vi "ihm_conv.vi"() -> ()   [LabVIEW 2014]
panel:
  out "out path":path
  out "nbrCmd":i32
  out "Array 2":u8[][](array[numeric]) format="%.0x"
  out "Numeric":i32
  out "length":i32
  out "reste":string
  out "parametre":string
  out "commande":string
  out "Lettre":string
  out "appended path":path
  out "text":string
  out "Array":string[](array[string])
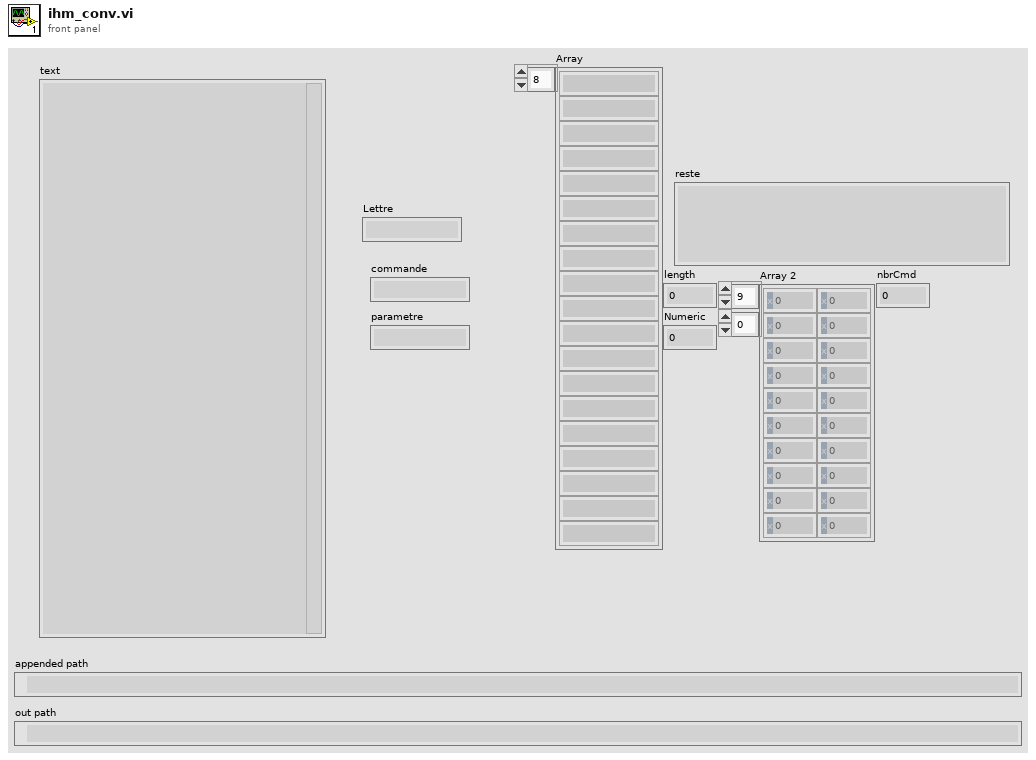
[diagram p1: front panel]
types:
  T1 = enum16{"open", "replace", "create", "open or create", "replace or create", "replace or create with confirmation"}
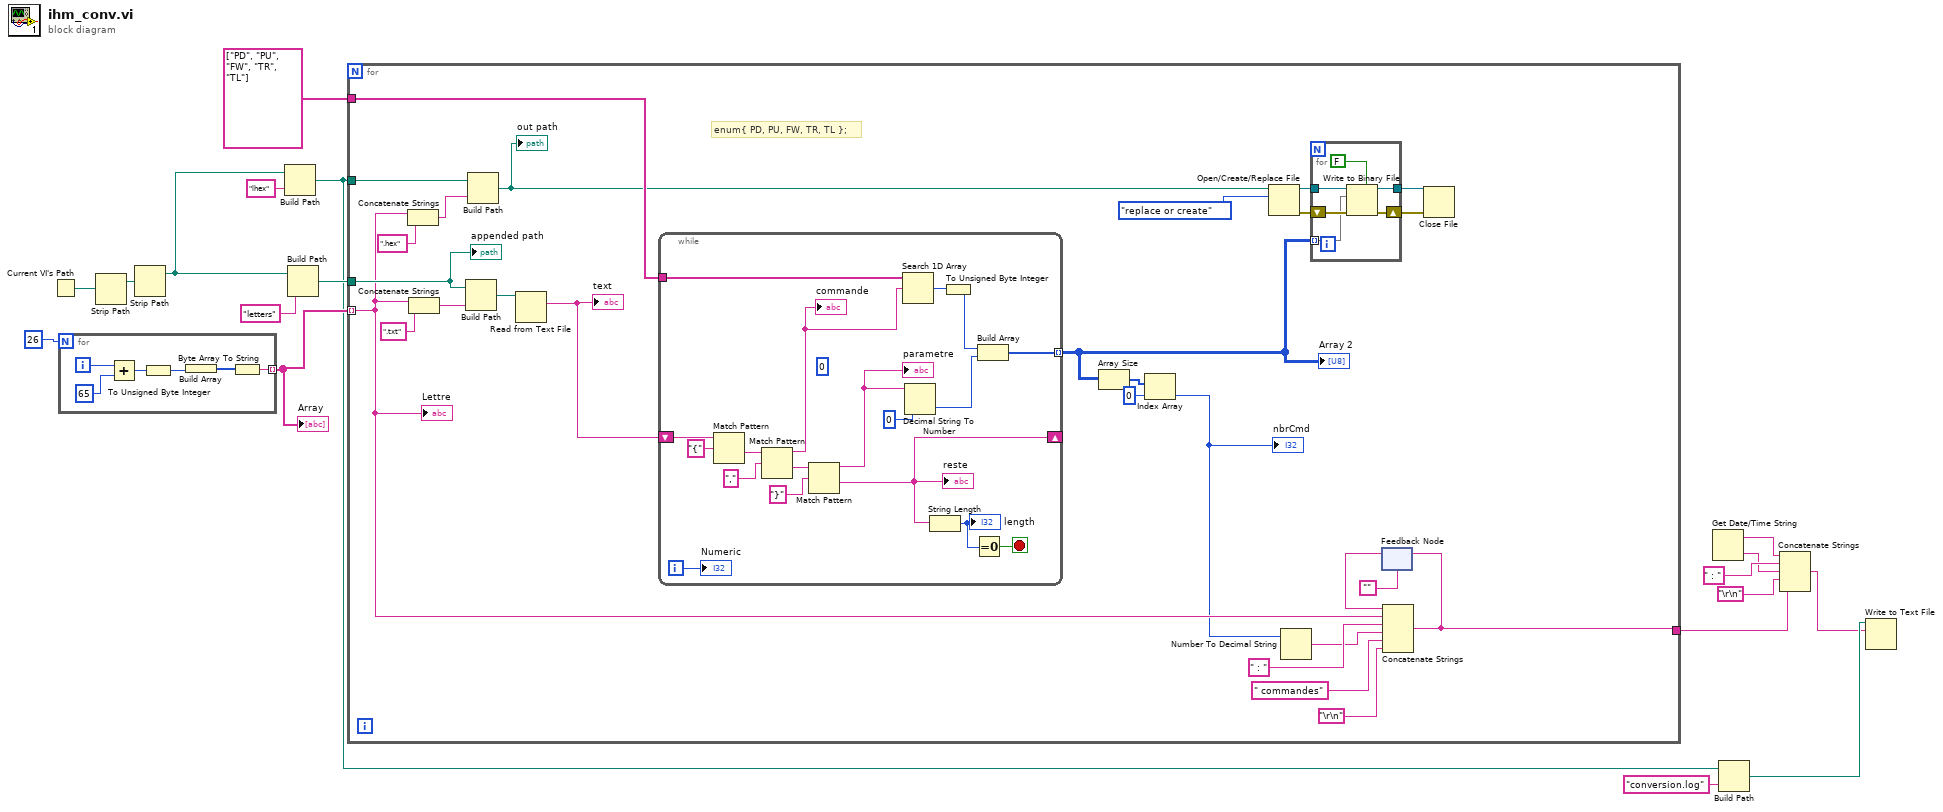
[diagram p0: block diagram]
diagram:
  n1 = Current VI's Path() -> (path=w17:path)
  n2 = for {
    N: 26 -> [_]
    tunnel: [w19] -> w15 mode=indexing
    i -> [w24]
    n3 = Add(x=w24, y=65) -> (x+y=w22:i32)
    n4 = To Unsigned Byte Integer(number=w22) -> (unsigned 8bit integer=w21:u8)
    n5 = Build Array(w21) -> (w20:u8[])
    n6 = Byte Array To String(unsigned byte array=w20) -> (string=w19:string)
  }
  "Array" <- w15
  n7 = Strip Path(path=w17) -> (stripped path=w13:path)  [unwired: 1 out]
  n8 = Strip Path(path=w13) -> (stripped path=w11:path)  [unwired: 1 out]
  n9 = Build Path(base path=w11, name or relative path="lhex") -> (appended path=w9:path)
  n10 = Build Path(base path=w11, name or relative path="letters") -> (appended path=w14:path)
  n11 = for {
    tunnel: w15 -> [w33] mode=indexing
    tunnel: w14 -> [w49]
    tunnel: w9 -> [w46]
    tunnel: string[] ["PD", "PU", "FW", "TR", "TL"] -> [w45]
    tunnel: [w28] -> w2
    # "enum{ PD, PU, FW, TR, TL };"
    n12 = Concatenate Strings(w33, ".hex" ("name or relative path")) -> (w41:string)
    n13 = Concatenate Strings(w33, ".txt" ("string")) -> (w47:string)
    n14 = Build Path(base path=w49, name or relative path=w47) -> (appended path=w51:path)
    n15 = Build Path(base path=w46, name or relative path=w41) -> (appended path=w40:path)
    "out path" <- w40
    n16 = Read from Text File(file (use dialog)=w51) -> (text=w50:string)  [unwired: 3 in, 3 out]
    "text" <- w50
    n17 = while {
      shift-right: [w69] -> _
      shift-left: w50 -> [w75]
      tunnel: [w62] -> w25 mode=indexing
      tunnel: w45 -> [w61]
      i -> [w68]
      stop <- w67 stop-if-true
      (unwired) u8 0
      n18 = Match Pattern(string=w75, regular expression="{") -> (after substring=w73:string)  [unwired: 1 in, 3 out]
      n19 = Match Pattern(string=w73, regular expression=",") -> (before substring=w60:string, after substring=w72:string)  [unwired: 1 in, 2 out]
      "commande" <- w60
      n20 = Match Pattern(string=w72, regular expression="}") -> (before substring=w65:string, after substring=w69:string)  [unwired: 1 in, 2 out]
      "parametre" <- w65
      "reste" <- w69
      n21 = Search 1D Array(1D array=w61, element=w60) -> (index of element=w59:i32)  [unwired: 1 in]
      n22 = Decimal String To Number(string=w65, default (0L)=u8 0) -> (number=w63:u8)  [unwired: 1 in, 1 out]
      n23 = String Length(string=w69) -> (length=w66:i32)
      "length" <- w66
      n24 = To Unsigned Byte Integer(number=w59) -> (unsigned 8bit integer=w58:u8)
      n25 = Equal To 0?(x=w66) -> (x = 0?=w67:bool)
      n26 = Build Array(w58, w63) -> (w62:u8[])
      "Numeric" <- w68
    }
    "Array 2" <- w25
    n27 = Array Size(array=w25) -> (size(s)=w44:i32[])
    n28 = Index Array(array=w44, index=0) -> (element=w26:i32)
    "nbrCmd" <- w26
    n29 = Open/Create/Replace File(file path (use dialog)=w40, operation (0:open)=T1."replace or create") -> (refnum out=w39:refnum<file>, error out=w38:errorcluster)  [unwired: 4 in, 1 out]
    n30 = Number To Decimal String(number=w26) -> (decimal integer string=w31:string)  [unwired: 1 in]
    n31 = for {
      tunnel: w25 -> [w55] mode=indexing
      shift-right: [w54] -> w37
      shift-left: w38 -> [w57]
      tunnel: w39 -> [w56]
      tunnel: [w53] -> w35
      n32 = Write to Binary File(file (use dialog)=w56, data=w55, error in=w57, 5:FALSE ("prepend array or string size? (T)")) -> (refnum out=w53:refnum<file>, error out=w54:errorcluster)  [unwired: 2 in, 1 out]
    }
    n33 = feedback #1("") -> (w34:string)
    n34 = Concatenate Strings(w34, w33, " : " ("string"), w31, " commandes" ("string"), "\r\n") -> (w28:string)
    n35 = feedback-in #1(w28) -> ()
    n36 = Close File(refnum=w35, error in=w37) -> ()  [unwired: 2 out]
    "appended path" <- w49
    "Lettre" <- w33
  }
  n37 = Get Date/Time String() -> (date string=w6:string, time string=w4:string)  [unwired: 3 in]
  n38 = Build Path(base path=w9, name or relative path="conversion.log") -> (appended path=w7:path)
  n39 = Concatenate Strings(w6, " : " ("string"), w4, "\r\n", w2) -> (w1:string)
  n40 = Write to Text File(file (use dialog)=w7, text=w1) -> ()  [unwired: 2 in, 3 out]
